vi "GearIntakeSingleton.vi"(8 "error in (no error)":errorcluster, 10 "Get/Set":enum16{"Get", "Set"}(ring), 11 "Gear Intake.lvclass":refnum<class "Gear Intake.lvclass">) -> (0 "error out":errorcluster, 3 "Gear Intake.lvclass":refnum<class "Gear Intake.lvclass">)   [LabVIEW 2016, in "Gear Intake.lvclass"]
uses:
  Gear Intake.lvclass
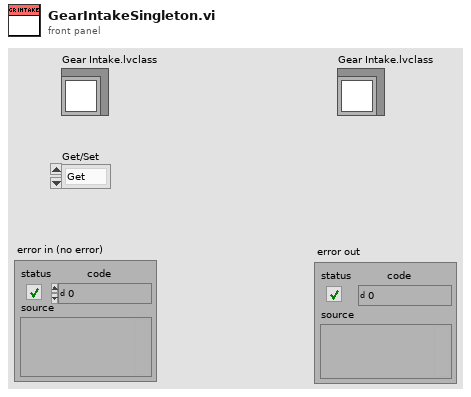
[diagram p1: front panel]
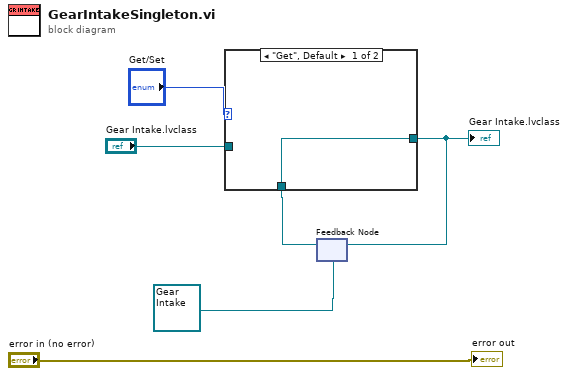
[diagram p0: block diagram]
diagram:
  n1 = feedback #1(refnum<class "Gear Intake.lvclass"> refnum ("Gear Intake.lvclass")) -> (w4:refnum<class "Gear Intake.lvclass">)
  n2 = case shown="\"Get\", Default" "Get/Set" {
    tunnel: "Gear Intake.lvclass" -> [_ _]
    tunnel: [w7 w8] -> w3
    tunnel: w4 -> [w7 w8]
    frame "Get", Default {
    }
    frame "Set" {
    }
  }
  "Gear Intake.lvclass" <- w3
  n3 = feedback-in #1(w3) -> ()
  "error out" <- "error in (no error)"
